vi "State String to Row Index.vi"(8 "error in (no error)":errorcluster, 10 "State String":string, 11 "StateMachine in":refnum<class "StateMachine.lvclass">) -> (0 "error out":errorcluster, 1 "State String found?":bool, 2 "Row Index":i32)   [LabVIEW 2018, in "State Machine.lvlib" / "StateMachine.lvclass"]
uses:
  StateMachine.lvclass
  StateMachine.lvclass/StateMachine.ctl
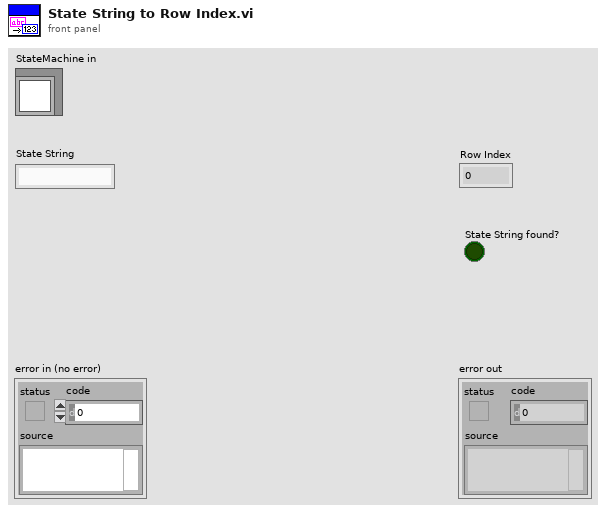
[diagram p1: front panel]
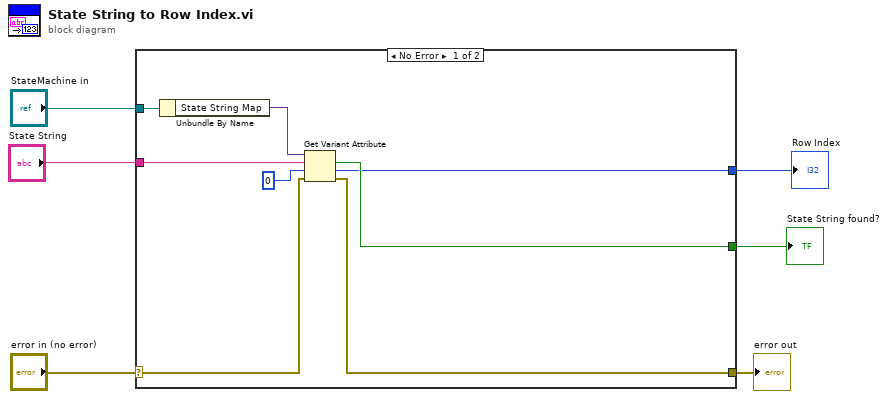
[diagram p0: block diagram]
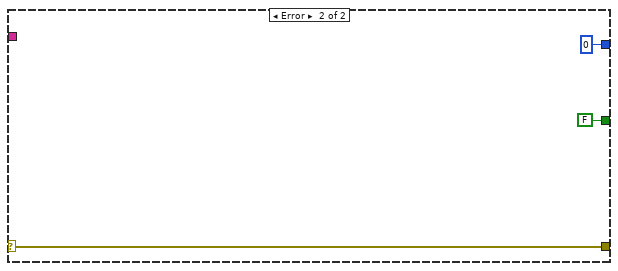
[diagram p2: hidden frame]
diagram:
  n1 = case shown="No Error" "error in (no error)" {
    selector: "error in (no error)" -> [w10 w17]
    tunnel: [w9 w17] -> w5
    tunnel: "StateMachine in" -> [w14 _]
    tunnel: "State String" -> [w12 _]
    tunnel: [w11 FALSE] -> w1
    tunnel: [w7 0] -> w2
    frame No Error {
      n2 = Unbundle By Name(w14) -> ("State String Map"=w13:variant)
      n3 = Get Variant Attribute(Variant=w13, name=w12, default value (empty Variant)=0, error in=w10) -> (found=w11:bool, value=w7:i32, error out=w9:errorcluster)  [unwired: 1 out]
    }
    frame Error {
    }
  }
  "error out" <- w5
  "Row Index" <- w2
  "State String found?" <- w1
